vi "Step 6 - Postprocessing.vi"() -> ()   [LabVIEW 2023]
doc: "Demonstrates how to use the DFD FXP MRate Postprocessing VI to convert the filtered signal from a fixed-point integer representation to readable engineering unit values."
uses:
  <vilib>/addons/Digital Filter Design/_Objects.llb/DFD Coef Norm Type.ctl
  <vilib>/addons/Digital Filter Design/FXPMRateSim.llb/DFD FXP MRate Simulation (DBL).vi
  <vilib>/addons/Digital Filter Design/FXPMRateSim.llb/DFD FXP MRate Postprocessing (I32, 1Ch).vi
  <vilib>/addons/Digital Filter Design/NI_DigFilterLicensed.lvlib
  <vilib>/Analysis/NI_AALBase.lvlib
panel:
  out "Filtered Signals":dbl[][](graph)
  # "Select Help>>Show Context Help and move the cursor over the VI icon for more information."
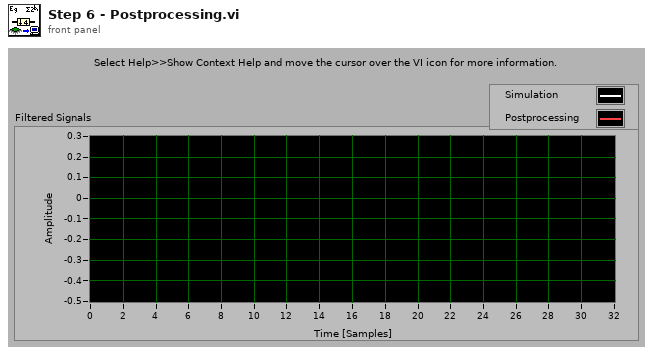
[diagram p1: front panel]
types:
  T1 = typedef "NI_DigFilterLicensed.lvlib/DFD Coef Norm Type.ctl" = enum16{"No Norm", "Time Domain 1-Norm", "Time Domain 2-Norm", "Time Domain Inf-Norm"}
  T2 = typedef "NI_DigFilterLicensed.lvlib/DFD Multirate Filter Obj.ctl" = cluster{"mMRate_Structure":enum16{"CIC", "FIR", "IIR", "Lattice"}, "mMRate_Mode":T3, "mMRate_Factor":i32, "mMRate_FIRParams":cluster{"mMRate_FIR_H":dbl[], "mMRate_FIR_IsNyquist?":bool, "mMRate_FIR_IsSymmetric?":bool}, "mMRate_CICParams":cluster{"mMRate_CIC_#Stage":i32, "mMRate_CIC_Lag":i32, "mMRate_CIC_Type":enum16{"Lowpass", "Highpass"}}, "mMRate_Order":i32, "mMRate_Version":string, "mMRate_Comments":string, "mMRate_RationalFactor":cluster{"mMRate_L":i32, "mMRate_M":i32}, "mMRate_Fs":dbl, "mMRate_Quantized?":bool, "mMRate_QFilterGain":dbl, "mMRate_CoefWl":i16, "mMRate_Scaling":cluster{"mMRate_ScaleByPowerOf2?":bool, "mMRate_ScaleType":T1}, "mMRate_InputWl":i16, "mMRate_OutputWl":i16, "mMRate_OutputMode":T4, "mMRate_MultMode":T5, "mMRate_BitPruning":bool, "mMRate_GainWl":i16, "mMRate_OutputFwl":i16, "mMRate_SumIwl":i16, "mMRate_InputIwl ":i16, "mMRate_SumWl":i16, "mMRate_CoefIwl":i16}
  T3 = typedef "NI_DigFilterLicensed.lvlib/DFD Multirate Mode.ctl" = i16
  T4 = typedef "NI_DigFilterLicensed.lvlib/DFD Round-off Mode.ctl" = enum16{"Nearest", "Truncation"}
  T5 = typedef "NI_DigFilterLicensed.lvlib/DFD FXP MRate Multiply Mode.ctl" = enum16{"Truncated", "Full"}
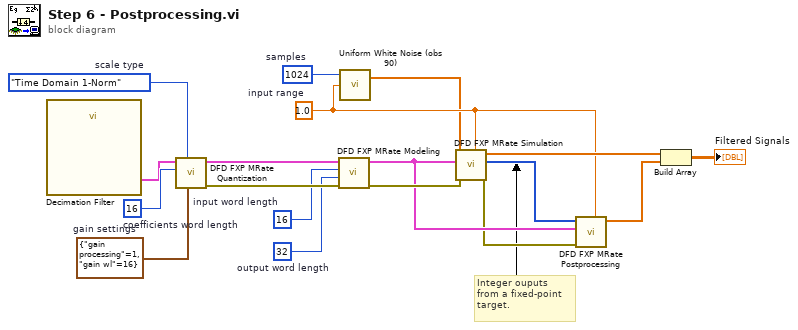
[diagram p0: block diagram]
diagram:
  w2 = i16 32  # output word length
  w3 = i16 16  # input word length
  w4 = i16 16  # coefficients word length
  w10 = cluster{"gain processing":u16, "gain wl":i16} {"gain processing"=1, "gain wl"=16}  # gain settings
  w11 = 1.0  # input range
  w15 = 1024  # samples
  w18 = DFD_Coef_Norm_Type."Time Domain 1-Norm"  # scale type
  # "Integer ouputs\nfrom a fixed-point\ntarget."
  n1 = call "Decimation Filter"() -> ("multirate filter out"=w1:T2)  [unwired: 11 out]
  n2 = call <vilib>:"DFD FXP MRate Quantization.vi"("gain settings"=w10, "scale type"=w18, "coefficients word length"=w4, "multirate filter in"=w1) -> ("error out"=w16:errorcluster, "multirate filter out"=w17:T2)  [unwired: 2 in, 4 out]
  n3 = call <vilib>:"DFD FXP MRate Modeling.vi"("error in (no error)"=w16, "output word length"=w2, "input word length"=w3, "multirate filter in"=w17) -> ("error out"=w9:errorcluster, "multirate filter out"=w8:T2)  [unwired: 4 in, 2 out]
  n4 = call <vilib>:"Uniform White Noise (obs 90).vi"("amplitude"=w11, "samples"=w15) -> ("uniform white noise"=w7:dbl[])  [unwired: 1 in, 1 out]
  n5 = call-poly <vilib>:"DFD FXP MRate Simulation.vi"("input range"=w11, "error in (no error)"=w9, "multirate filter"=w8, "signal in"=w7) -> ("error out"=w6:errorcluster, "integer signal out"=w5:i32[], "DBL signal out"=w13:dbl[])  [unwired: 1 in, 4 out]
  n6 = call-poly <vilib>:"DFD FXP MRate Postprocessing.vi"("input range"=w11, "error in (no error)"=w6, "multirate filter"=w8, "signal in"=w5) -> ("signal out"=w12:dbl[])  [unwired: 1 in, 6 out]
  n7 = Build Array(w13, w12) -> (→"Filtered Signals":dbl[][])
